vi "find indices.vi"(1 "value to compare":string="1", 2 "search array":string[](array[string])) -> (0 "indices":i32[](array[numeric]))   [LabVIEW 2013]
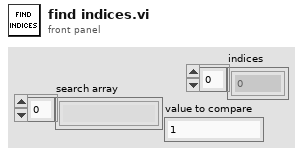
[diagram p1: front panel]
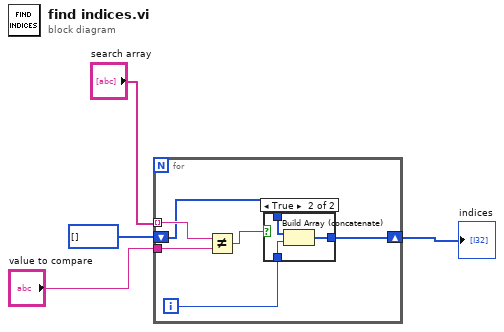
[diagram p0: block diagram]
diagram:
  n1 = for {
    tunnel: "search array" -> [w10] mode=indexing
    shift-right: [w6] -> w1
    shift-left: i32[] [] -> [w7]
    tunnel: "value to compare" -> [w5]
    i -> [w8]
    n2 = Not Equal?(x=w10, y=w5) -> (x != y?=w9:bool)
    n3 = case shown="True" w9 {
      tunnel: w8 -> [_ w14]
      tunnel: [w11 w13] -> w6
      tunnel: w7 -> [w11 w12]
      frame False {
      }
      frame True {
        n4 = Build Array (concatenate)(w12, w14) -> (w13:i32[])
      }
    }
  }
  "indices" <- w1
